vi "UR_message_generator.vi"(3 "Object orientation":dbl, 4 "Obejct CoM Y":dbl, 5 "Object CoM X":dbl, 6 "Obejct length":dbl) -> (0 "Task Out":string, 1 "UR message":string, 2 "Tool Out":string)   [LabVIEW 2022 SP3]
doc: "Convertes object coordinates, length and orientation to a message for the UR"
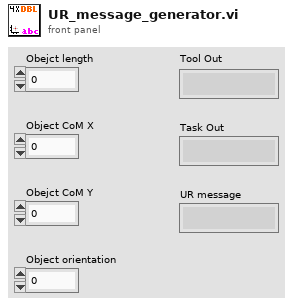
[diagram p1: front panel]
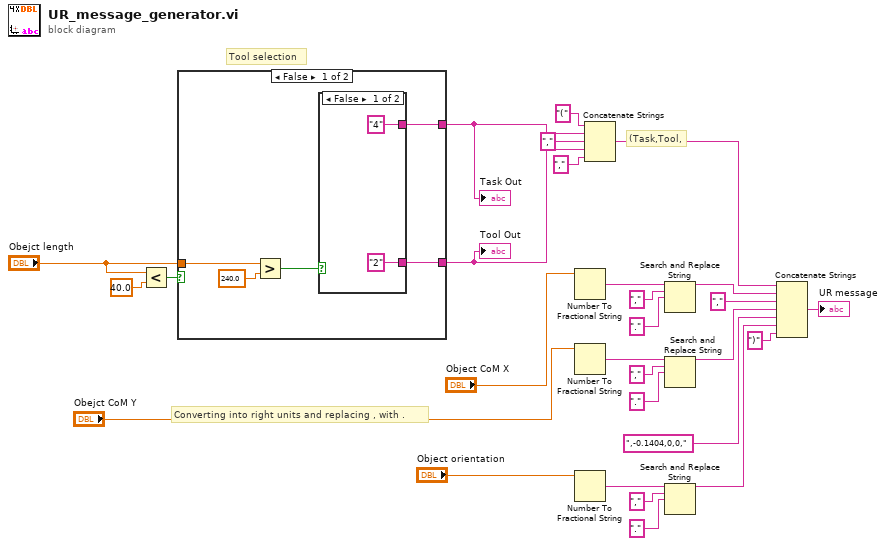
[diagram p0: block diagram]
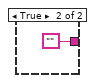
[diagram p2: hidden frame]
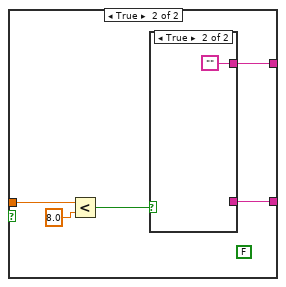
[diagram p3: hidden frame]
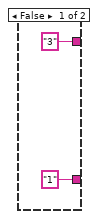
[diagram p4: hidden frame]
diagram:
  # "(Task,Tool,"
  # "Converting into right units and replacing , with ."
  # "Tool selection"
  n1 = Less?(x="Obejct length", y=40.0) -> (x < y?=w9:bool)
  n2 = case shown="False" w9 {
    tunnel: [w33 w37] -> w2
    tunnel: "Obejct length" -> [w31 w39]
    tunnel: [w29 w38] -> w5
    frame False {
      n3 = Greater?(x=w31, y=240.0) -> (0:w32:bool)
      n4 = case shown="False" w32 {
        tunnel: ["2" _] -> w33
        tunnel: ["4" ""] -> w29
        frame False {
        }
        frame True {
        }
      }
    }
    frame True {
      (unwired) FALSE
      n5 = Less?(x=w39, y=8.0) -> (x < y?=w41:bool)
      n6 = case shown="True" w41 {
        tunnel: ["3" ""] -> w38
        tunnel: ["1" _] -> w37
        frame False {
        }
        frame True {
        }
      }
    }
  }
  "Tool Out" <- w2
  "Task Out" <- w5
  n7 = Number To Fractional String(number="Object CoM X") -> (F-format string=w11:string)  [unwired: 3 in]
  n8 = Number To Fractional String(number="Obejct CoM Y") -> (F-format string=w17:string)  [unwired: 3 in]
  n9 = Number To Fractional String(number="Object orientation") -> (F-format string=w13:string)  [unwired: 3 in]
  n10 = Concatenate Strings("(" ("string"), w5, "," ("string"), w2, "," ("string")) -> (w3:string)
  n11 = Search and Replace String(input string=w11, search string=",", replace string="." ("replace string (\"\")")) -> (result string=w20:string)  [unwired: 5 in, 3 out]
  n12 = Search and Replace String(input string=w17, search string=",", replace string="." ("replace string (\"\")")) -> (result string=w16:string)  [unwired: 5 in, 3 out]
  n13 = Search and Replace String(input string=w13, search string=",", replace string="." ("replace string (\"\")")) -> (result string=w12:string)  [unwired: 5 in, 3 out]
  n14 = Concatenate Strings(w3, w20, "," ("string"), w16, ",-0.1404,0,0," ("string"), w12, ")" ("string")) -> (→"UR message":string)
